vi "Autonomous Independent.vi"() -> ()   [LabVIEW 2015]
doc: "This VI is called when autonomous begins, and will automatically be terminated when autonomous ends. You can carry out timed or sensor driven robot movement independently without needing to return to the caller."
uses:
  <vilib>/Rock Robotics/WPI/Utilities/WPI_GetSetVariantRefNum.vi
  <vilib>/Rock Robotics/Network Tables/NT Write Numeric Array.vi
  <vilib>/Rock Robotics/Network Tables/NT Read Boolean.vi
  <vilib>/Rock Robotics/WPI/RobotDrive/WPI_RobotDriveArcadeDrive_Standard(NoSaturation).vi
  <vilib>/Rock Robotics/Network Tables/NT Write Boolean.vi
  <vilib>/Rock Robotics/Network Tables/NT Write Number.vi
  <vilib>/Rock Robotics/Network Tables/NT Read Number.vi
panel:
  in  "Ticks to Turn Right":i32
  in  "To goto the edge of the goal":i32=10
  in  "Value to Raise to.":dbl=70.0
  out "POT Sensor Meter 2":dbl(knob) scale=78.0..98.0
  out "POT Sensor Value 2":dbl
  in  "Ticks to Turn Left":i32=8
  in  "Distance to goto pass the Defence":i32=55
  in  "Ticks to Drive forwad close to the turnning Point":i32=63
  in  "Desides the Distance for Loop 1":i32=16
  out "VAR-Storage-1":dbl
  out "Low Switch":bool
  out "High Switch":bool
  out "POT Sensor Meter":dbl(knob) scale=78.0..98.0
  out "POT Sensor Value":dbl
  # "Also This value is the \nTotal amount of ticks not Turns!\n\nSo 6 Ticks EQU 1 Full Turn."
  # "Remeber to Right Click:\nData Operatoins -> Make Current Value Default"
  # "LOOP 1 - LOOP 1 - LOOP 1 - LOOP 1 - LOOP 1 - LOOP 1 - LOOP 1 - LOOP 1 - LOOP 1 - LOOP 1 - LOOP 1"
  # "DRIVE PAST THE DEFENCE"
  # "LOOP 2  - LOOP 2  - LOOP 2  - LOOP 2  - LOOP 2  - LOOP 2 -  LOOP 2 - LOOP 2  - LOOP 2  - LOOP 2 - LOOP 2"
  # "THIS IS TO DRIVE PAST THE DEFENCE AND TRY TO SHOT"
  # "LOOP 3  - LOOP 3  - LOOP 3  - LOOP 3  - LOOP 3  - LOOP 3  - LOOP 3  - LOOP 3  - LOOP 3  - LOOP 3 - LOOP 3"
  # "Go Past the Defence."
  # "Be sure to right-click and choose Data Operations>>Make Current Value default if you want to save the array values with the VI"
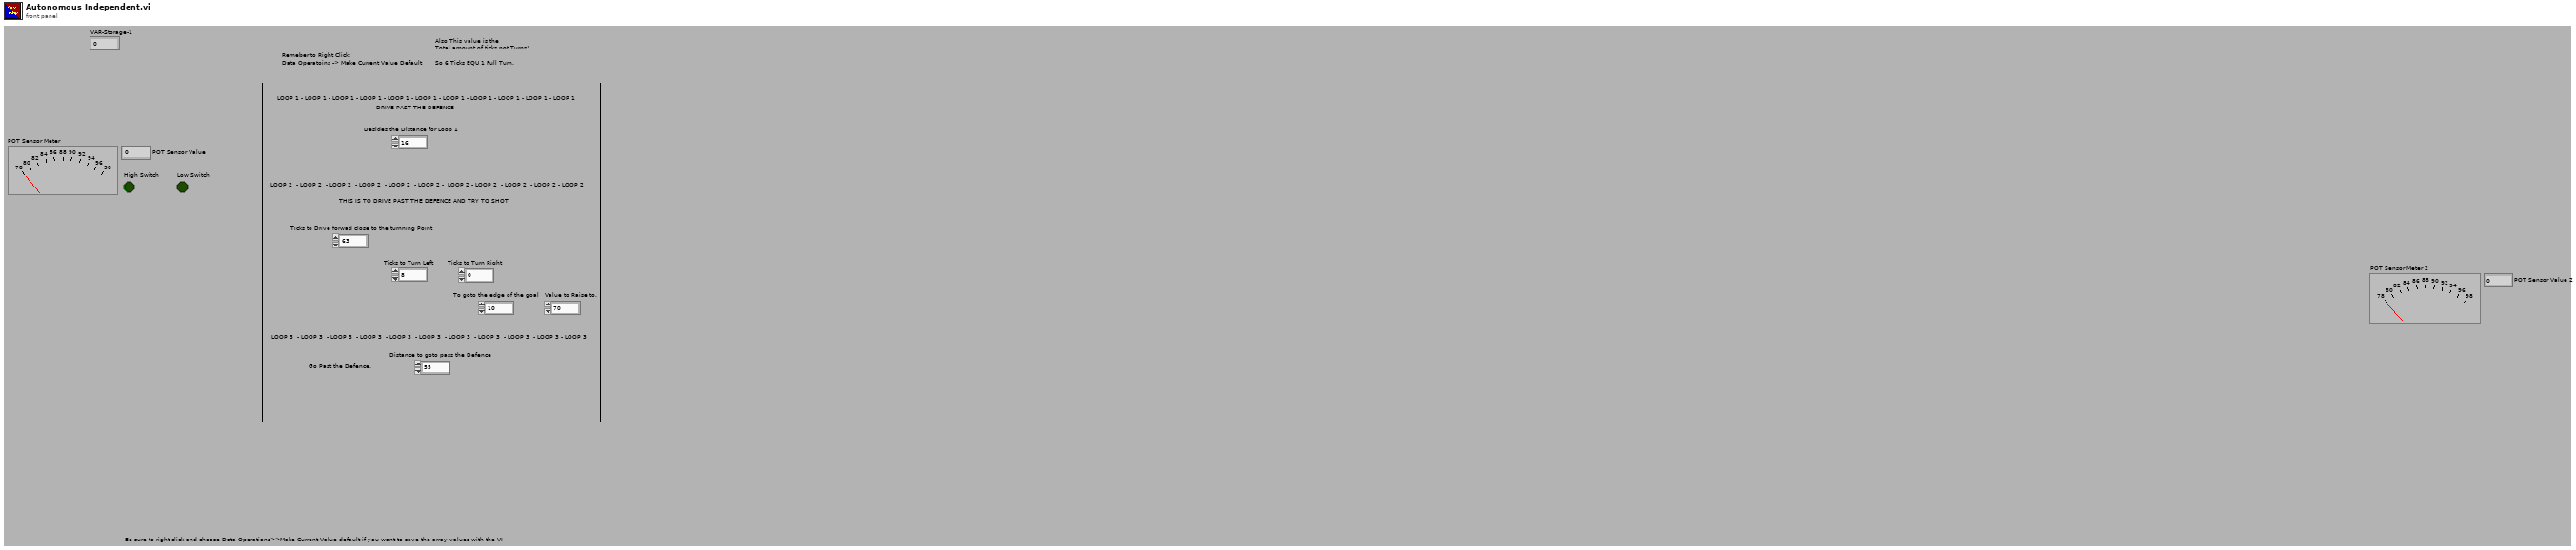
[diagram p1: front panel]
types:
  T1 = typedef "WPI_JoystickDevRef.ctl" = cluster{"Device":T2}
  T2 = typedef "WPI_JoystickDeviceEnum.ctl" = enum16{"USB 0", "USB 1", "USB 2", "USB 3", "USB 4", "USB 5"}
  T3 = typedef "WPI_CounterDevRef.ctl" = cluster{"DevStatus":errorcluster, "CntIndex":T4}
  T4 = typedef "FPGA_CounterCtrSystemIndex.ctl" = enum8{"Ctr 0", "Ctr 1", "Ctr 2", "Ctr 3", "Ctr 4", "Ctr 5", "Ctr 6", "Ctr 7", "Invalid"}
  T5 = typedef "WPI_RobotDriveDevRef.ctl" = cluster{"DevStatus":errorcluster, "Motors[]":T6[], "Square Inputs":bool, "Max Output":dbl}
  T6 = typedef "WPI_MotorControlDeviceRef.ctl" = cluster{"DeviceStatus":errorcluster, "Type":T7, "PWM":cluster{"PWM Channel":T8, "DeadBand":T9}, "CAN":cluster{"Device Number":u8, "Control Mode":T10, "Semaphore":T11, "Max Vout":dbl, "TalonSRX Control Mode":T12}, "Invert":bool}
  T7 = typedef "WPI_MotorControlType.ctl" = enum16{"PWM", "CAN", "CANTalonSRX"}
  T8 = typedef "FPGA_DIOPWMChannel.ctl" = enum8{"PWM 0", "PWM 1", "PWM 2", "PWM 3", "PWM 4", "PWM 5", "PWM 6", "PWM 7", "PWM 8", "PWM 9", "PWM MXP 0", "PWM MXP 1", "PWM MXP 2", "PWM MXP 3", "PWM MXP 4", "PWM MXP 5", "PWM MXP 6", "PWM MXP 7", "PWM MXP 8", "PWM MXP 9", "Invalid"}
  T9 = typedef "WPI_PWMDeadband.ctl" = cluster{"Name":string, "maxPositivePwm":i32, "minPositivePwm":i32, "centerPwm":i32, "maxNegativePwm":i32, "minNegativePwm":i32, "angularRange":u16}
  T10 = typedef "WPI_CANJaguar_ControlMode.ctl" = enum8{"Percent VBus", "Current", "Speed", "Position", "Voltage"}
  T11 = typedef "Semaphore RefNum" = refnum<k1>
  T12 = typedef "WPI_CANTalonSRX_APIControlMode.ctl" = enum8{"Percent VBus", "Speed", "Position", "Slave", "Unchanged / Invalid", "Voltage Compensation", "Current", "Motion Profile"}
  T13 = typedef "WPI_SwitchDevRef.ctl" = cluster{"DevStatus":errorcluster, "DIO Channel":T14, "CntIndex":T4, "Normally Closed":bool}
  T14 = typedef "FPGA_DIOChannel.ctl" = enum8{"DIO 0", "DIO 1", "DIO 2", "DIO 3", "DIO 4", "DIO 5", "DIO 6", "DIO 7", "DIO 8", "DIO 9", "DIO MXP 0", "DIO MXP 1", "DIO MXP 2", "DIO MXP 3", "DIO MXP 4", "DIO MXP 5", "DIO MXP 6", "DIO MXP 7", "DIO MXP 8", "DIO MXP 9", "DIO MXP 10", "DIO MXP 11", "DIO MXP 12", "DIO MXP 13", "DIO MXP 14", "DIO MXP 15", "Invalid"}
  T15 = typedef "WPI_PotentiometerDevRef.ctl" = cluster{"DevStatus":errorcluster, "Analog Channel":T16, "Invert Output":bool}
  T16 = typedef "FPGA_AIChannel.ctl" = enum8{"AI 0", "AI 1", "AI 2", "AI 3", "AI MXP 0", "AI MXP 1", "AI MXP 2", "AI MXP 3", "Invalid"}
  T17 = typedef "WPI_ServoDeviceRef.ctl" = cluster{"DeviceStatus":errorcluster, "PWM Channel":T8, "DeadBand":T9}
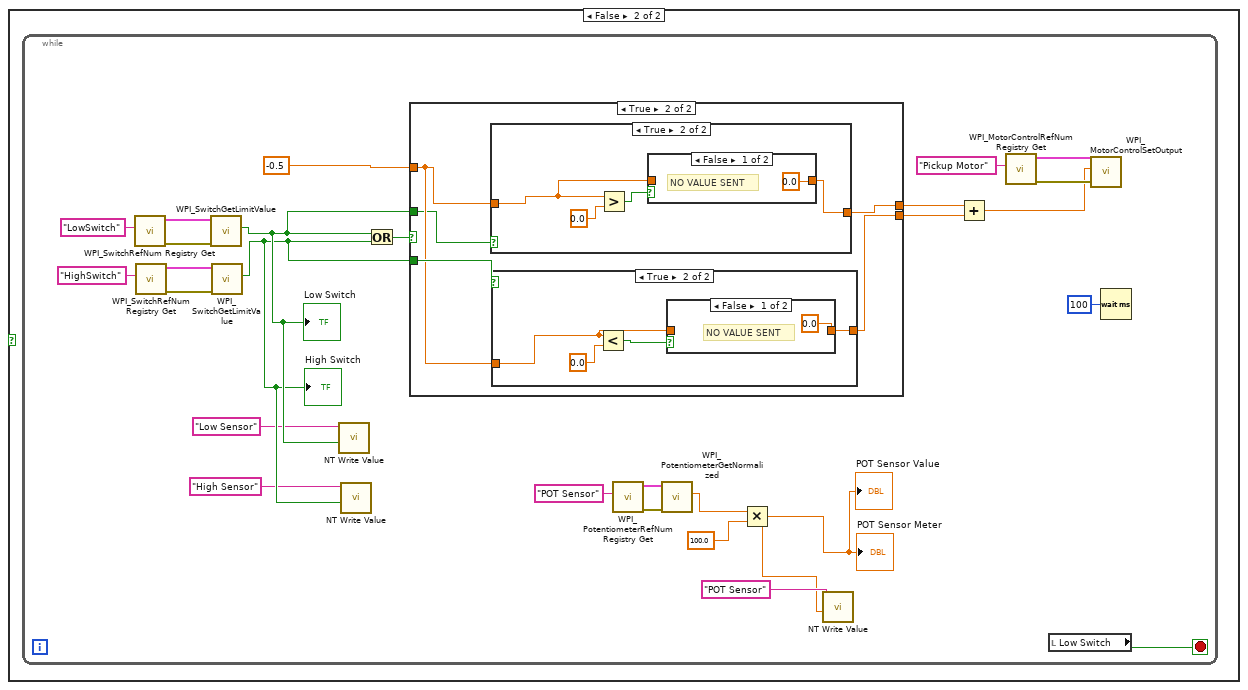
[diagram p2: hidden frame]
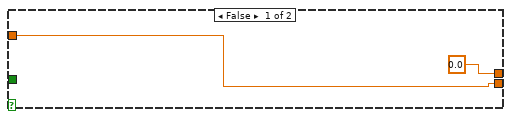
[diagram p3: hidden frame]
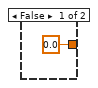
[diagram p4: hidden frame]
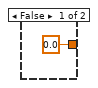
[diagram p6: hidden frame]
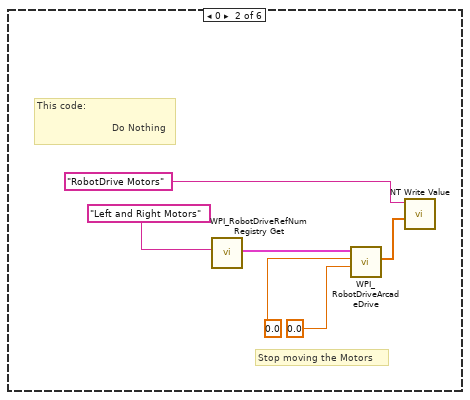
[diagram p9: hidden frame]
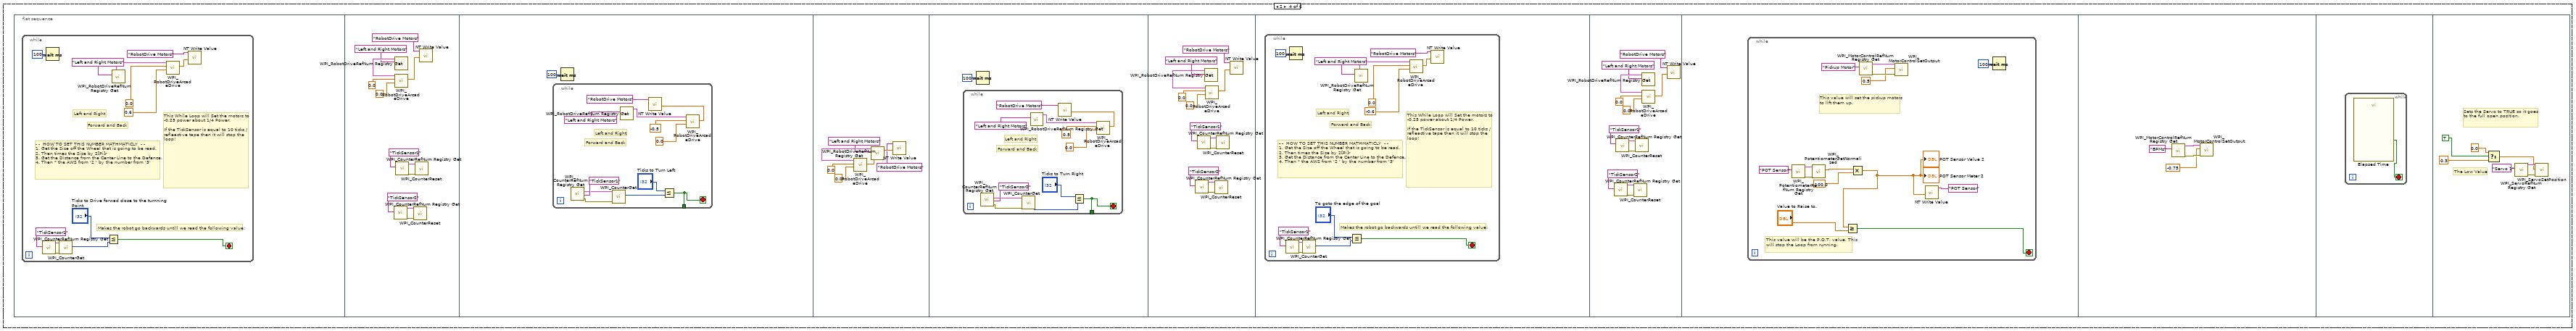
[diagram p10: hidden frame]
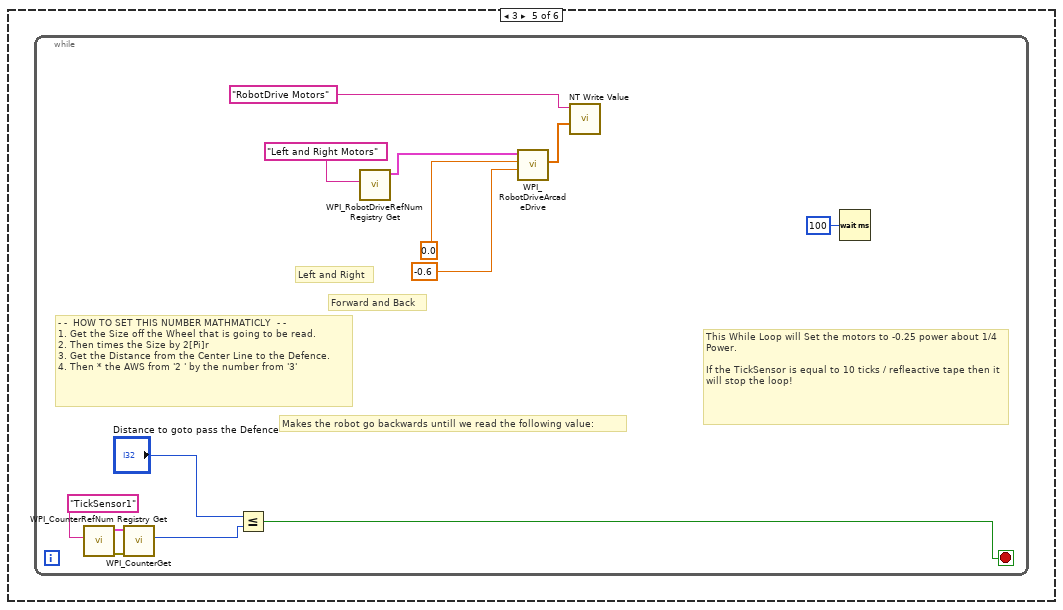
[diagram p11: hidden frame]
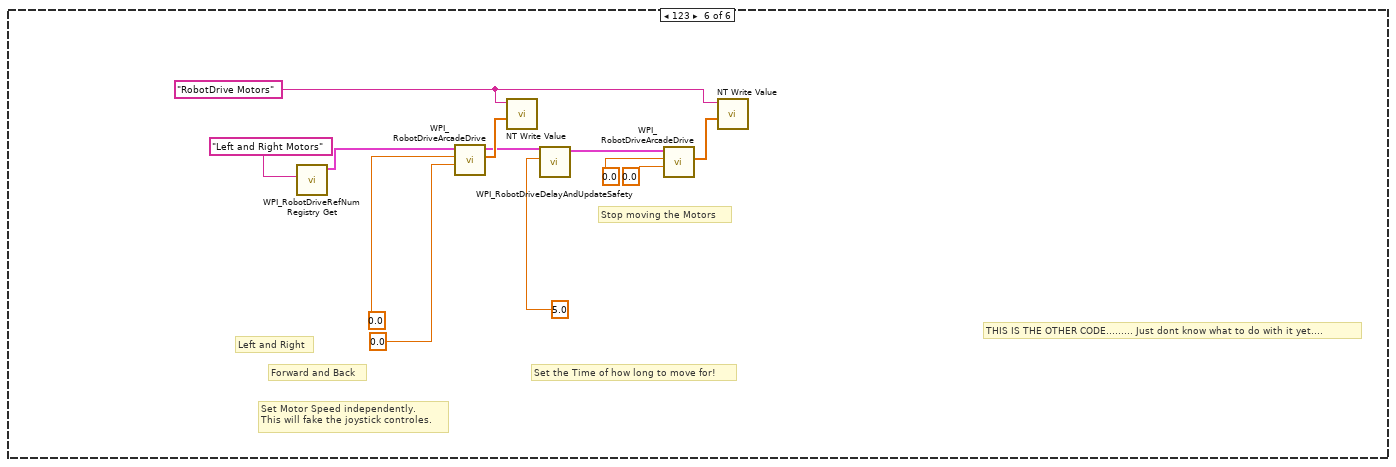
[diagram p12: hidden frame]
diagram:
  (unwired) "This function is run in parallel when the autonomous period begins. It will be terminated automatically when the period ends.\n\nNote that all Driver Station inputs are automatically latched and will not change once auto begins."
  # "Every 20ms, report that we are running autonomous\ncode. Loop will abort the same time as the VI."
  # "This gives you the joystick value\nthat is often the throttle"
  # "This tells you the driver position\nand alliance color"
  n1 = while {
    stop <- FALSE stop-if-true
    n2 = call <vilib>:"WPI_DriverStationReport Robot Code State.vi"("Autonomous"=TRUE) -> ()  [unwired: 10 in, 1 out]
    n3 = Wait (ms)(milliseconds to wait=u32 20) -> ()  [unwired: 1 out]
  }
  n4 = call <vilib>:"WPI_DriverStationGet Alliance Info.vi"() -> ()  [unwired: 12 out]
  n5 = call <vilib>:"WPI_JoystickRefNum Registry Get.vi"("refnum name"="Joystick 0") -> ("JoystickDevRef"=w5:T1)  [unwired: 1 in, 9 out]
  n6 = call-poly <vilib>:"NT Read Value.vi"("Name"="Auto Selector") -> ()  [unwired: 9 in, 2 out]
  n7 = call <vilib>:"WPI_JoystickGetValues.vi"("JoystickDevRef"=w5) -> ("Axes"=w3:dbl[])  [unwired: 6 in, 4 out]
  n8 = call-poly <vilib>:"NT Write Value.vi"("Numeric Array"=w3, "Name"="Joystick 0/Axes") -> ()  [unwired: 9 in, 1 out]
  n9 = Index Array(array=w3, index=2) -> ()  [unwired: 1 out]
  n10 = flat-sequence {
    frame #0 {
      n11 = call <vilib>:"WPI_CounterRefNum Registry Get.vi"("refnum name"="TickSensor1") -> ("error out"=w15:errorcluster, "CounterDevRef"=w16:T3)  [unwired: 9 in]
      n12 = call <vilib>:"WPI_RobotDriveRefNum Registry Get.vi"("refnum name"="Left and Right Motors") -> ("RobotDriveDevRef"=w17:T5)  [unwired: 1 in, 9 out]
      n13 = call <vilib>:"WPI_CounterReset.vi"("error in (no error)"=w15, "CounterDevRef in"=w16) -> ()  [unwired: 8 in, 2 out]
      n14 = call <vilib>:"WPI_MotorControlRefNum Registry Get.vi"("refnum name"="BPMs") -> ("error out"=w12:errorcluster, "MotorControlDevRef"=w11:T6)  [unwired: 9 in]
      n15 = call <vilib>:"WPI_MotorControlSetOutput.vi"("error in (no error)"=w12, "Output"=0.0, "MotorControlDevRef"=w11) -> ()  [unwired: 6 in, 3 out]
      n16 = call <vilib>:"WPI_CounterRefNum Registry Get.vi"("refnum name"="TickSensor2") -> ("error out"=w24:errorcluster, "CounterDevRef"=w23:T3)  [unwired: 9 in]
      n17 = call <vilib>:"WPI_CounterReset.vi"("error in (no error)"=w24, "CounterDevRef in"=w23) -> ()  [unwired: 8 in, 2 out]
      n18 = call-poly <vilib>:"WPI_RobotDriveArcadeDrive.vi"("Y axis value"=0.0 ("X axis value"), "X axis value"=0.0, "RobotDriveDevRef"=w17) -> ("Motor Values"=w19:dbl[])  [unwired: 1 in, 7 out]
      n19 = call-poly <vilib>:"NT Write Value.vi"("Numeric Array"=w19, "Name"="RobotDrive Motors") -> ()  [unwired: 9 in, 1 out]
    }
    frame #1 {
      n20 = call-poly <vilib>:"NT Read Value.vi"("Default Value"=FALSE, "Name"="DisableLowerOnStart") -> ()  [unwired: 8 in, 2 out]
      n21 = case shown="True" TRUE {
        frame True {
          # "Puts a Wait for this program so it will make the loop not do anything."
          # "Disabling the Shoot from dropping down automaticly. By Default the code will automaticly put down the shoot. If the Button on the drive station is pressed then it will automaticly skip the loop and prevent the bukket from going down."
          n22 = Wait (ms)(milliseconds to wait=u32 0) -> ()  [unwired: 1 out]
        }
        frame False {
          n23 = while {
            stop <- w31 stop-if-true
            n24 = call <vilib>:"WPI_SwitchRefNum Registry Get.vi"("refnum name"="LowSwitch") -> ("error out"=w54:errorcluster, "SwitchDevRef"=w55:T13)  [unwired: 9 in]
            n25 = call <vilib>:"WPI_SwitchRefNum Registry Get.vi"("refnum name"="HighSwitch") -> ("error out"=w51:errorcluster, "SwitchDevRef"=w52:T13)  [unwired: 9 in]
            n26 = call <vilib>:"WPI_SwitchGetLimitValue.vi"("error in (no error)"=w54, "SwitchDevRef"=w55) -> ("Switch Pressed"=w39:bool)  [unwired: 7 in, 2 out]
            "Low Switch" <- w39
            n27 = call <vilib>:"WPI_SwitchGetLimitValue.vi"("error in (no error)"=w51, "SwitchDevRef"=w52) -> ("Switch Pressed"=w38:bool)  [unwired: 7 in, 2 out]
            "High Switch" <- w38
            n28 = call-poly <vilib>:"NT Write Value.vi"("Boolean"=w39, "Name"="Low Sensor") -> ()  [unwired: 9 in, 1 out]
            n29 = call-poly <vilib>:"NT Write Value.vi"("Boolean"=w38, "Name"="High Sensor") -> ()  [unwired: 9 in, 1 out]
            n30 = Or(x=w39, y=w38) -> (x .or. y?=w56:bool)
            n31 = case shown="True" w56 {
              tunnel: w39 -> [_ w61]
              tunnel: w38 -> [_ w63]
              tunnel: -0.5 ("Axes[1]") -> [w57 w62]
              tunnel: [0.0 ("Axes[1]") w60] -> w45
              tunnel: [w57 w59] -> w44
              frame False {
              }
              frame True {
                n32 = case shown="True" w61 {
                  tunnel: w62 -> [_ w73]
                  tunnel: [0.0 ("Axes[1]") w72] -> w60
                  frame False {
                  }
                  frame True {
                    n33 = Greater?(x=w73, y=0.0) -> (0:w74:bool)
                    n34 = case shown="False" w74 {
                      tunnel: [0.0 ("Axes[1]") w77] -> w72
                      tunnel: w73 -> [_ w77]
                      frame False {
                        # "NO VALUE SENT"
                      }
                      frame True {
                      }
                    }
                  }
                }
                n35 = case shown="True" w63 {
                  tunnel: w62 -> [_ w65]
                  tunnel: [0.0 ("Axes[1]") w66] -> w59
                  frame False {
                  }
                  frame True {
                    n36 = Less?(x=w65, y=0.0) -> (x < y?=w67:bool)
                    n37 = case shown="False" w67 {
                      tunnel: [0.0 ("Axes[1]") w70] -> w66
                      tunnel: w65 -> [_ w70]
                      frame False {
                        # "NO VALUE SENT"
                      }
                      frame True {
                      }
                    }
                  }
                }
              }
            }
            n38 = call <vilib>:"WPI_PotentiometerRefNum Registry Get.vi"("refnum name"="POT Sensor") -> ("error out"=w43:errorcluster, "PotDevRef"=w42:T15)  [unwired: 9 in]
            n39 = call <vilib>:"WPI_PotentiometerGetNormalized.vi"("error in"=w43, "PotDevRef"=w42) -> ("Normalized Value"=w35:dbl)  [unwired: 7 in, 2 out]
            n40 = Multiply(x=w35, y=100.0) -> (x*y=w33:dbl)
            "POT Sensor Value" <- w33
            "POT Sensor Meter" <- w33
            n41 = call-poly <vilib>:"NT Write Value.vi"("Numeric"=w33, "Name"="POT Sensor") -> ()  [unwired: 9 in, 1 out]
            n42 = Add(x=w45, y=w44) -> (x+y=w46:dbl)
            n43 = call <vilib>:"WPI_MotorControlRefNum Registry Get.vi"("refnum name"="Pickup Motor") -> ("error out"=w49:errorcluster, "MotorControlDevRef"=w48:T6)  [unwired: 9 in]
            n44 = local read "Low Switch"() -> (w31:bool)
            n45 = call <vilib>:"WPI_MotorControlSetOutput.vi"("error in (no error)"=w49, "Output"=w46, "MotorControlDevRef"=w48) -> ()  [unwired: 6 in, 3 out]
            n46 = Wait (ms)(milliseconds to wait=u32 100) -> ()  [unwired: 1 out]
          }
        }
      }
    }
    frame #2 {
      # "This tells you the autonomous selected\nfrom the dashboard"
      n47 = call-poly <vilib>:"NT Read Value.vi"("Name"="AutoModeSelector") -> ("Numeric"=w79:dbl)  [unwired: 9 in, 1 out]
      n48 = Wait (ms)(milliseconds to wait=u32 20) -> ()  [unwired: 1 out]
      n49 = case shown="1" w79 {
        frame Default {
          # "You can put your main auto here, or you can right-click on the case and make any\nother frame be the default case."
          # "This is the frame that will execute if no selection is made, or if it is not recognized"
        }
        frame 0 {
          # "Stop moving the Motors"
          # "This code:\n                   \n                         Do Nothing"
          n50 = call <vilib>:"WPI_RobotDriveRefNum Registry Get.vi"("refnum name"="Left and Right Motors") -> ("RobotDriveDevRef"=w81:T5)  [unwired: 1 in, 9 out]
          n51 = call-poly <vilib>:"WPI_RobotDriveArcadeDrive.vi"("Y axis value"=0.0 ("X axis value"), "X axis value"=0.0, "RobotDriveDevRef"=w81) -> ("Motor Values"=w85:dbl[])  [unwired: 1 in, 7 out]
          n52 = call-poly <vilib>:"NT Write Value.vi"("Numeric Array"=w85, "Name"="RobotDrive Motors") -> ()  [unwired: 9 in, 1 out]
        }
        frame 1 {
          n53 = while {
            stop <- w96 stop-if-true
            # "NEGATIVE IS FORWARD!!!!\nPOSATIVE IS BACKWARD!!!"
            # "- -  HOW TO SET THIS NUMBER MATHMATICLY  - - \n1. Get the Size off the Wheel that is going to be read.\n2. Then times the Size by 2[Pi]r\n3. Get the Distance from the Center Line to the Defence.\n4. Then * the AWS from '2 ' by the number from '3'"
            # "Makes the robot go backwards untill we read the following value:"
            # "This While Loop will Set the motors to -0.25 power about 1/4 Power.\n\nIf the TickSensor is equal to 10 ticks / refleactive tape then it will stop the loop!"
            # "Forward and Back"
            # "Left and Right"
            n54 = call <vilib>:"WPI_CounterRefNum Registry Get.vi"("refnum name"="TickSensor1") -> ("error out"=w98:errorcluster, "CounterDevRef"=w97:T3)  [unwired: 9 in]
            n55 = call <vilib>:"WPI_CounterGet.vi"("error in (no error)"=w98, "CounterDevRef in"=w97) -> ("Value"=w88:i32)  [unwired: 4 in, 5 out]
            n56 = Less Or Equal?(x="Desides the Distance for Loop 1", y=w88) -> (x <= y?=w96:bool)
            n57 = call <vilib>:"WPI_RobotDriveRefNum Registry Get.vi"("refnum name"="Left and Right Motors") -> ("RobotDriveDevRef"=w95:T5)  [unwired: 1 in, 9 out]
            n58 = call-poly <vilib>:"WPI_RobotDriveArcadeDrive.vi"("Y axis value"=-0.6 ("X axis value"), "X axis value"=0.0, "RobotDriveDevRef"=w95) -> ("Motor Values"=w93:dbl[])  [unwired: 1 in, 7 out]
            n59 = call-poly <vilib>:"NT Write Value.vi"("Numeric Array"=w93, "Name"="RobotDrive Motors") -> ()  [unwired: 9 in, 1 out]
            n60 = Wait (ms)(milliseconds to wait=u32 100) -> ()  [unwired: 1 out]
          }
        }
        frame 2 {
          n61 = flat-sequence {
            frame #0 {
              n62 = while {
                stop <- w109 stop-if-true
                # "- -  HOW TO SET THIS NUMBER MATHMATICLY  - - \n1. Get the Size off the Wheel that is going to be read.\n2. Then times the Size by 2[Pi]r\n3. Get the Distance from the Center Line to the Defence.\n4. Then * the AWS from '2 ' by the number from '3'"
                # "Makes the robot go backwards untill we read the following value:"
                # "This While Loop will Set the motors to -0.25 power about 1/4 Power.\n\nIf the TickSensor is equal to 10 ticks / refleactive tape then it will stop the loop!"
                # "Forward and Back"
                # "Left and Right"
                n63 = call <vilib>:"WPI_CounterRefNum Registry Get.vi"("refnum name"="TickSensor1") -> ("error out"=w111:errorcluster, "CounterDevRef"=w110:T3)  [unwired: 9 in]
                n64 = Wait (ms)(milliseconds to wait=u32 100) -> ()  [unwired: 1 out]
                n65 = call <vilib>:"WPI_CounterGet.vi"("error in (no error)"=w111, "CounterDevRef in"=w110) -> ("Value"=w101:i32)  [unwired: 4 in, 5 out]
                n66 = Less Or Equal?(x="Ticks to Drive forwad close to the turnning Point", y=w101) -> (x <= y?=w109:bool)
                n67 = call <vilib>:"WPI_RobotDriveRefNum Registry Get.vi"("refnum name"="Left and Right Motors") -> ("RobotDriveDevRef"=w108:T5)  [unwired: 1 in, 9 out]
                n68 = call-poly <vilib>:"WPI_RobotDriveArcadeDrive.vi"("Y axis value"=0.6 ("X axis value"), "X axis value"=0.0, "RobotDriveDevRef"=w108) -> ("Motor Values"=w106:dbl[])  [unwired: 1 in, 7 out]
                n69 = call-poly <vilib>:"NT Write Value.vi"("Numeric Array"=w106, "Name"="RobotDrive Motors") -> ()  [unwired: 9 in, 1 out]
              }
            }
            frame #1 {
              n70 = call <vilib>:"WPI_CounterRefNum Registry Get.vi"("refnum name"="TickSensor2") -> ("error out"=w120:errorcluster, "CounterDevRef"=w119:T3)  [unwired: 9 in]
              n71 = call <vilib>:"WPI_RobotDriveRefNum Registry Get.vi"("refnum name"="Left and Right Motors") -> ("RobotDriveDevRef"=w118:T5)  [unwired: 1 in, 9 out]
              n72 = call-poly <vilib>:"WPI_RobotDriveArcadeDrive.vi"("Y axis value"=0.0 ("X axis value"), "X axis value"=0.0, "RobotDriveDevRef"=w118) -> ("Motor Values"=w116:dbl[])  [unwired: 1 in, 7 out]
              n73 = call <vilib>:"WPI_CounterRefNum Registry Get.vi"("refnum name"="TickSensor1") -> ("error out"=w123:errorcluster, "CounterDevRef"=w122:T3)  [unwired: 9 in]
              n74 = call <vilib>:"WPI_CounterReset.vi"("error in (no error)"=w120, "CounterDevRef in"=w119) -> ()  [unwired: 8 in, 2 out]
              n75 = call <vilib>:"WPI_CounterReset.vi"("error in (no error)"=w123, "CounterDevRef in"=w122) -> ()  [unwired: 8 in, 2 out]
              n76 = call-poly <vilib>:"NT Write Value.vi"("Numeric Array"=w116, "Name"="RobotDrive Motors") -> ()  [unwired: 9 in, 1 out]
            }
            frame #2 {
              n77 = while {
                tunnel: [w126] -> _
                stop <- w126 stop-if-true
                # "Forward and Back"
                # "Left and Right"
                n78 = call <vilib>:"WPI_CounterRefNum Registry Get.vi"("refnum name"="TickSensor1") -> ("error out"=w136:errorcluster, "CounterDevRef"=w135:T3)  [unwired: 9 in]
                n79 = call <vilib>:"WPI_CounterGet.vi"("error in (no error)"=w136, "CounterDevRef in"=w135) -> ("Value"=w129:i32)  [unwired: 4 in, 5 out]
                n80 = call <vilib>:"WPI_RobotDriveRefNum Registry Get.vi"("refnum name"="Left and Right Motors") -> ("RobotDriveDevRef"=w134:T5)  [unwired: 1 in, 9 out]
                n81 = Less Or Equal?(x="Ticks to Turn Left", y=w129) -> (x <= y?=w126:bool)
                n82 = call-poly <vilib>:"WPI_RobotDriveArcadeDrive.vi"("Y axis value"=0.0 ("X axis value"), "X axis value"=-0.5, "RobotDriveDevRef"=w134) -> ("Motor Values"=w133:dbl[])  [unwired: 1 in, 7 out]
                n83 = call-poly <vilib>:"NT Write Value.vi"("Numeric Array"=w133, "Name"="RobotDrive Motors") -> ()  [unwired: 9 in, 1 out]
              }
              n84 = Wait (ms)(milliseconds to wait=u32 100) -> ()  [unwired: 1 out]
            }
            frame #3 {
              n85 = call <vilib>:"WPI_RobotDriveRefNum Registry Get.vi"("refnum name"="Left and Right Motors") -> ("RobotDriveDevRef"=w138:T5)  [unwired: 1 in, 9 out]
              n86 = call-poly <vilib>:"WPI_RobotDriveArcadeDrive.vi"("Y axis value"=0.0 ("X axis value"), "X axis value"=0.0, "RobotDriveDevRef"=w138) -> ("Motor Values"=w140:dbl[])  [unwired: 1 in, 7 out]
              n87 = call-poly <vilib>:"NT Write Value.vi"("Numeric Array"=w140, "Name"="RobotDrive Motors") -> ()  [unwired: 9 in, 1 out]
            }
            frame #4 {
              n88 = while {
                tunnel: [w145] -> _
                stop <- w145 stop-if-true
                # "Forward and Back"
                # "Left and Right"
                n89 = call <vilib>:"WPI_CounterRefNum Registry Get.vi"("refnum name"="TickSensor2") -> ("error out"=w155:errorcluster, "CounterDevRef"=w154:T3)  [unwired: 9 in]
                n90 = call <vilib>:"WPI_CounterGet.vi"("error in (no error)"=w155, "CounterDevRef in"=w154) -> ("Value"=w148:i32)  [unwired: 4 in, 5 out]
                n91 = call <vilib>:"WPI_RobotDriveRefNum Registry Get.vi"("refnum name"="Left and Right Motors") -> ("RobotDriveDevRef"=w153:T5)  [unwired: 1 in, 9 out]
                n92 = Less Or Equal?(x="Ticks to Turn Right", y=w148) -> (x <= y?=w145:bool)
                n93 = call-poly <vilib>:"WPI_RobotDriveArcadeDrive.vi"("Y axis value"=0.0 ("X axis value"), "X axis value"=0.5, "RobotDriveDevRef"=w153) -> ("Motor Values"=w152:dbl[])  [unwired: 1 in, 7 out]
                n94 = call-poly <vilib>:"NT Write Value.vi"("Numeric Array"=w152, "Name"="RobotDrive Motors") -> ()  [unwired: 9 in, 1 out]
              }
              n95 = Wait (ms)(milliseconds to wait=u32 100) -> ()  [unwired: 1 out]
            }
            frame #5 {
              n96 = call <vilib>:"WPI_CounterRefNum Registry Get.vi"("refnum name"="TickSensor2") -> ("error out"=w164:errorcluster, "CounterDevRef"=w163:T3)  [unwired: 9 in]
              n97 = call <vilib>:"WPI_CounterRefNum Registry Get.vi"("refnum name"="TickSensor1") -> ("error out"=w167:errorcluster, "CounterDevRef"=w166:T3)  [unwired: 9 in]
              n98 = call <vilib>:"WPI_RobotDriveRefNum Registry Get.vi"("refnum name"="Left and Right Motors") -> ("RobotDriveDevRef"=w162:T5)  [unwired: 1 in, 9 out]
              n99 = call-poly <vilib>:"WPI_RobotDriveArcadeDrive.vi"("Y axis value"=0.0 ("X axis value"), "X axis value"=0.0, "RobotDriveDevRef"=w162) -> ("Motor Values"=w160:dbl[])  [unwired: 1 in, 7 out]
              n100 = call <vilib>:"WPI_CounterReset.vi"("error in (no error)"=w164, "CounterDevRef in"=w163) -> ()  [unwired: 8 in, 2 out]
              n101 = call <vilib>:"WPI_CounterReset.vi"("error in (no error)"=w167, "CounterDevRef in"=w166) -> ()  [unwired: 8 in, 2 out]
              n102 = call-poly <vilib>:"NT Write Value.vi"("Numeric Array"=w160, "Name"="RobotDrive Motors") -> ()  [unwired: 9 in, 1 out]
            }
            frame #6 {
              n103 = while {
                stop <- w178 stop-if-true
                # "- -  HOW TO SET THIS NUMBER MATHMATICLY  - - \n1. Get the Size off the Wheel that is going to be read.\n2. Then times the Size by 2[Pi]r\n3. Get the Distance from the Center Line to the Defence.\n4. Then * the AWS from '2 ' by the number from '3'"
                # "Makes the robot go backwards untill we read the following value:"
                # "This While Loop will Set the motors to -0.25 power about 1/4 Power.\n\nIf the TickSensor is equal to 10 ticks / refleactive tape then it will stop the loop!"
                # "Forward and Back"
                # "Left and Right"
                n104 = call <vilib>:"WPI_CounterRefNum Registry Get.vi"("refnum name"="TickSensor1") -> ("error out"=w180:errorcluster, "CounterDevRef"=w179:T3)  [unwired: 9 in]
                n105 = Wait (ms)(milliseconds to wait=u32 100) -> ()  [unwired: 1 out]
                n106 = call <vilib>:"WPI_CounterGet.vi"("error in (no error)"=w180, "CounterDevRef in"=w179) -> ("Value"=w170:i32)  [unwired: 4 in, 5 out]
                n107 = Less Or Equal?(x="To goto the edge of the goal", y=w170) -> (x <= y?=w178:bool)
                n108 = call <vilib>:"WPI_RobotDriveRefNum Registry Get.vi"("refnum name"="Left and Right Motors") -> ("RobotDriveDevRef"=w177:T5)  [unwired: 1 in, 9 out]
                n109 = call-poly <vilib>:"WPI_RobotDriveArcadeDrive.vi"("Y axis value"=-0.6 ("X axis value"), "X axis value"=0.0, "RobotDriveDevRef"=w177) -> ("Motor Values"=w175:dbl[])  [unwired: 1 in, 7 out]
                n110 = call-poly <vilib>:"NT Write Value.vi"("Numeric Array"=w175, "Name"="RobotDrive Motors") -> ()  [unwired: 9 in, 1 out]
              }
            }
            frame #7 {
              n111 = call <vilib>:"WPI_CounterRefNum Registry Get.vi"("refnum name"="TickSensor2") -> ("error out"=w189:errorcluster, "CounterDevRef"=w188:T3)  [unwired: 9 in]
              n112 = call <vilib>:"WPI_CounterRefNum Registry Get.vi"("refnum name"="TickSensor1") -> ("error out"=w192:errorcluster, "CounterDevRef"=w191:T3)  [unwired: 9 in]
              n113 = call <vilib>:"WPI_CounterReset.vi"("error in (no error)"=w189, "CounterDevRef in"=w188) -> ()  [unwired: 8 in, 2 out]
              n114 = call <vilib>:"WPI_CounterReset.vi"("error in (no error)"=w192, "CounterDevRef in"=w191) -> ()  [unwired: 8 in, 2 out]
              n115 = call <vilib>:"WPI_RobotDriveRefNum Registry Get.vi"("refnum name"="Left and Right Motors") -> ("RobotDriveDevRef"=w187:T5)  [unwired: 1 in, 9 out]
              n116 = call-poly <vilib>:"WPI_RobotDriveArcadeDrive.vi"("Y axis value"=0.0 ("X axis value"), "X axis value"=0.0, "RobotDriveDevRef"=w187) -> ("Motor Values"=w185:dbl[])  [unwired: 1 in, 7 out]
              n117 = call-poly <vilib>:"NT Write Value.vi"("Numeric Array"=w185, "Name"="RobotDrive Motors") -> ()  [unwired: 9 in, 1 out]
            }
            frame #8 {
              n118 = while {
                stop <- w201 stop-if-true
                # "This value will set the pickup motors to lift them up."
                # "This value will be the P.O.T. value. This will stop the Loop from running."
                n119 = call <vilib>:"WPI_PotentiometerRefNum Registry Get.vi"("refnum name"="POT Sensor") -> ("error out"=w207:errorcluster, "PotDevRef"=w206:T15)  [unwired: 9 in]
                n120 = call <vilib>:"WPI_PotentiometerGetNormalized.vi"("error in"=w207, "PotDevRef"=w206) -> ("Normalized Value"=w203:dbl)  [unwired: 7 in, 2 out]
                n121 = Multiply(x=w203, y=100.0) -> (x*y=w200:dbl)
                "POT Sensor Value 2" <- w200
                "POT Sensor Meter 2" <- w200
                n122 = Greater Or Equal?(x=w200, y="Value to Raise to.") -> (x >= y?=w201:bool)
                n123 = call <vilib>:"WPI_MotorControlRefNum Registry Get.vi"("refnum name"="Pickup Motor") -> ("error out"=w199:errorcluster, "MotorControlDevRef"=w198:T6)  [unwired: 9 in]
                n124 = call <vilib>:"WPI_MotorControlSetOutput.vi"("error in (no error)"=w199, "Output"=0.5, "MotorControlDevRef"=w198) -> ()  [unwired: 6 in, 3 out]
                n125 = call-poly <vilib>:"NT Write Value.vi"("Numeric"=w200, "Name"="POT Sensor") -> ()  [unwired: 9 in, 1 out]
                n126 = Wait (ms)(milliseconds to wait=u32 100) -> ()  [unwired: 1 out]
              }
            }
            frame #9 {
              n127 = call <vilib>:"WPI_MotorControlRefNum Registry Get.vi"("refnum name"="BPMs") -> ("error out"=w210:errorcluster, "MotorControlDevRef"=w209:T6)  [unwired: 9 in]
              n128 = call <vilib>:"WPI_MotorControlSetOutput.vi"("error in (no error)"=w210, "Output"=-0.75, "MotorControlDevRef"=w209) -> ()  [unwired: 6 in, 3 out]
            }
            frame #10 {
              n129 = while {
                stop <- w212 stop-if-true
                n130 = call "Elapsed Time"() -> ("Time has Elapsed"=w212:bool)  [unwired: 12 in, 7 out]
              }
            }
            frame #11 {
              # "Sets the Servo to TRUE so it goes to the full open position."
              # "The Low Value"
              n131 = Select(t=0.0, s=TRUE, f=0.3) -> (s? t:f=w214:dbl)
              n132 = call <vilib>:"WPI_ServoRefNum Registry Get.vi"("refnum name"="Servo 1") -> ("error out"=w218:errorcluster, "ServoDeviceRef"=w217:T17)  [unwired: 9 in]
              n133 = call <vilib>:"WPI_ServoSetPosition.vi"("error in (no error)"=w218, "Position"=w214, "ServoDeviceRef"=w217) -> ()  [unwired: 7 in, 2 out]
            }
          }
        }
        frame 3 {
          n134 = while {
            stop <- w229 stop-if-true
            # "- -  HOW TO SET THIS NUMBER MATHMATICLY  - - \n1. Get the Size off the Wheel that is going to be read.\n2. Then times the Size by 2[Pi]r\n3. Get the Distance from the Center Line to the Defence.\n4. Then * the AWS from '2 ' by the number from '3'"
            # "Makes the robot go backwards untill we read the following value:"
            # "This While Loop will Set the motors to -0.25 power about 1/4 Power.\n\nIf the TickSensor is equal to 10 ticks / refleactive tape then it will stop the loop!"
            # "Forward and Back"
            # "Left and Right"
            n135 = call <vilib>:"WPI_CounterRefNum Registry Get.vi"("refnum name"="TickSensor1") -> ("error out"=w231:errorcluster, "CounterDevRef"=w230:T3)  [unwired: 9 in]
            n136 = call <vilib>:"WPI_CounterGet.vi"("error in (no error)"=w231, "CounterDevRef in"=w230) -> ("Value"=w221:i32)  [unwired: 4 in, 5 out]
            n137 = Less Or Equal?(x="Distance to goto pass the Defence", y=w221) -> (x <= y?=w229:bool)
            n138 = call <vilib>:"WPI_RobotDriveRefNum Registry Get.vi"("refnum name"="Left and Right Motors") -> ("RobotDriveDevRef"=w228:T5)  [unwired: 1 in, 9 out]
            n139 = call-poly <vilib>:"WPI_RobotDriveArcadeDrive.vi"("Y axis value"=-0.6 ("X axis value"), "X axis value"=0.0, "RobotDriveDevRef"=w228) -> ("Motor Values"=w226:dbl[])  [unwired: 1 in, 7 out]
            n140 = call-poly <vilib>:"NT Write Value.vi"("Numeric Array"=w226, "Name"="RobotDrive Motors") -> ()  [unwired: 9 in, 1 out]
            n141 = Wait (ms)(milliseconds to wait=u32 100) -> ()  [unwired: 1 out]
          }
        }
        frame 123 {
          w243 = "RobotDrive Motors" ("Name")
          # "THIS IS THE OTHER CODE......... Just dont know what to do with it yet...."
          # "Forward and Back"
          # "Left and Right"
          # "Set Motor Speed independently.\nThis will fake the joystick controles."
          # "Set the Time of how long to move for!"
          # "Stop moving the Motors"
          n142 = call <vilib>:"WPI_RobotDriveRefNum Registry Get.vi"("refnum name"="Left and Right Motors") -> ("RobotDriveDevRef"=w244:T5)  [unwired: 1 in, 9 out]
          n143 = call-poly <vilib>:"WPI_RobotDriveArcadeDrive.vi"("Y axis value"=0.0 ("X axis value"), "X axis value"=0.0, "RobotDriveDevRef"=w244) -> ("Motor Values"=w242:dbl[], "RobotDriveDevRef"=w236:T5)  [unwired: 1 in, 6 out]
          n144 = call-poly <vilib>:"NT Write Value.vi"("Numeric Array"=w242, "Name"=w243) -> ()  [unwired: 9 in, 1 out]
          n145 = call <vilib>:"WPI_RobotDriveDelayAndUpdateSafety.vi"("Delay (s)"=5.0, "RobotDriveDevRef"=w236) -> ("RobotDriveDevRef 2"=w235:T5)  [unwired: 8 in, 1 out]
          n146 = call-poly <vilib>:"WPI_RobotDriveArcadeDrive.vi"("Y axis value"=0.0 ("X axis value"), "X axis value"=0.0, "RobotDriveDevRef"=w235) -> ("Motor Values"=w241:dbl[])  [unwired: 1 in, 7 out]
          n147 = call-poly <vilib>:"NT Write Value.vi"("Numeric Array"=w241, "Name"=w243) -> ()  [unwired: 9 in, 1 out]
        }
      }
    }
    frame #3 {
      n148 = call <vilib>:"WPI_RobotDriveRefNum Registry Get.vi"("refnum name"="Left and Right Motors") -> ("RobotDriveDevRef"=w255:T5)  [unwired: 1 in, 9 out]
      n149 = call <vilib>:"WPI_MotorControlRefNum Registry Get.vi"("refnum name"="BPMs") -> ("error out"=w247:errorcluster, "MotorControlDevRef"=w246:T6)  [unwired: 9 in]
      n150 = call <vilib>:"WPI_CounterRefNum Registry Get.vi"("refnum name"="TickSensor2") -> ("error out"=w253:errorcluster, "CounterDevRef"=w254:T3)  [unwired: 9 in]
      n151 = call <vilib>:"WPI_CounterRefNum Registry Get.vi"("refnum name"="TickSensor1") -> ("error out"=w250:errorcluster, "CounterDevRef"=w251:T3)  [unwired: 9 in]
      n152 = call <vilib>:"WPI_MotorControlSetOutput.vi"("error in (no error)"=w247, "Output"=0.0, "MotorControlDevRef"=w246) -> ()  [unwired: 6 in, 3 out]
      n153 = call <vilib>:"WPI_CounterReset.vi"("error in (no error)"=w253, "CounterDevRef in"=w254) -> ()  [unwired: 8 in, 2 out]
      n154 = call <vilib>:"WPI_CounterReset.vi"("error in (no error)"=w250, "CounterDevRef in"=w251) -> ()  [unwired: 8 in, 2 out]
      n155 = call-poly <vilib>:"WPI_RobotDriveArcadeDrive.vi"("Y axis value"=0.0 ("X axis value"), "X axis value"=0.0, "RobotDriveDevRef"=w255) -> ("Motor Values"=w257:dbl[])  [unwired: 1 in, 7 out]
      n156 = call-poly <vilib>:"NT Write Value.vi"("Numeric Array"=w257, "Name"="RobotDrive Motors") -> ()  [unwired: 9 in, 1 out]
    }
  }
